vi "get_single_acq_wrapper.vi"(8 "error in (no error)":errorcluster, 11 "_camera in":refnum<class "_camera.lvclass">) -> (0 "error out":errorcluster, 1 "trigger":dbl[][](array[numeric]), 2 "raw data":i32[][][](array[numeric]), 3 "_camera out":refnum<class "_camera.lvclass">)   [LabVIEW 2019, in "_camera.lvlib" / "_camera.lvclass"]
uses:
  _camera.lvclass
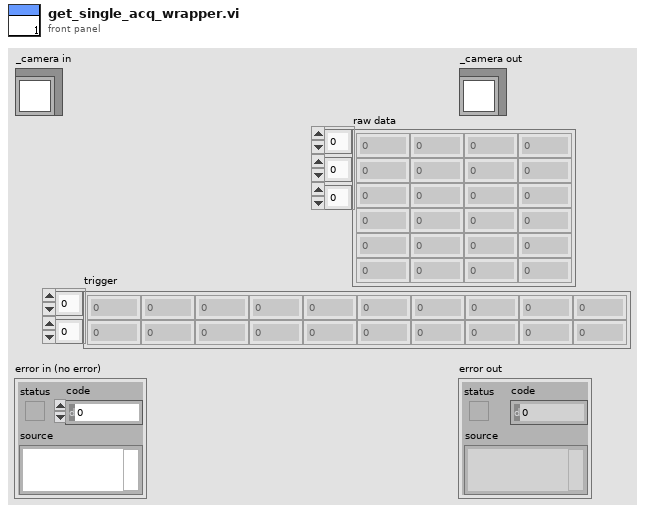
[diagram p1: front panel]
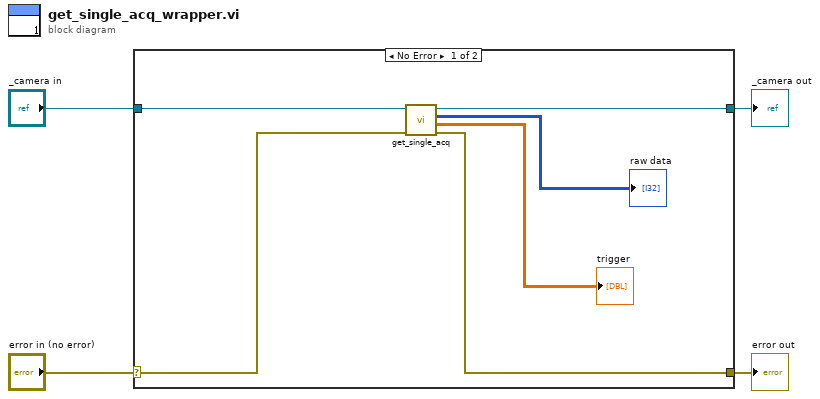
[diagram p0: block diagram]
diagram:
  n1 = case shown="No Error" "error in (no error)" {
    selector: "error in (no error)" -> [w8 w12]
    tunnel: [w7 w12] -> w3
    tunnel: [w9 w11] -> w1
    tunnel: "_camera in" -> [w10 w11]
    frame No Error {
      n2 = call-dynamic "get_single_acq.vi"("error in (no error)"=w8, "_camera in"=w10) -> ("error out"=w7:errorcluster, "trigger"=→"trigger":dbl[][], "raw data"=→"raw data":i32[][][], "_camera out"=w9:refnum<class "_camera.lvclass">)  [unwired: 6 in]
    }
    frame Error {
    }
  }
  "error out" <- w3
  "_camera out" <- w1
